vi "FOR.vi"() -> ()   [LabVIEW 2020]
panel:
  out "Numeric 2":i32
  out "Array 2":i32[](array[numeric])
  out "Array":i32[](array[numeric])
  out "Tank":u8(slide) scale=0.0..50.0
  in  "Numeric":i32
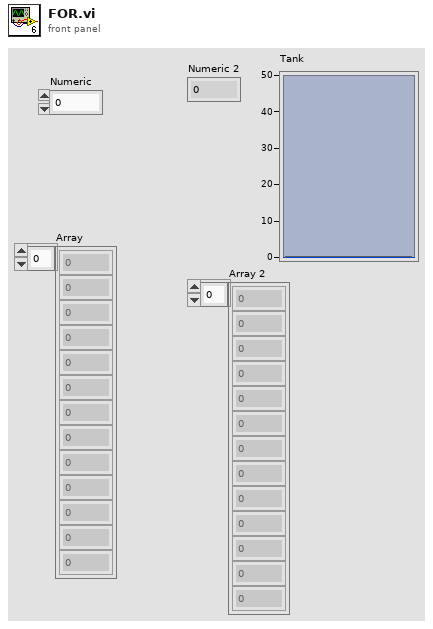
[diagram p1: front panel]
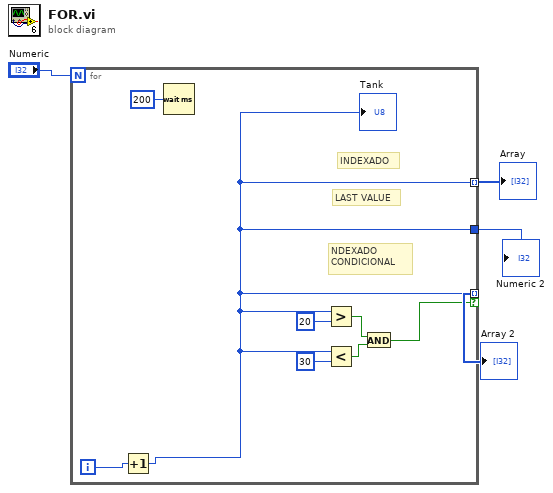
[diagram p0: block diagram]
diagram:
  n1 = for {
    N: "Numeric" -> [_]
    tunnel: [w5] -> w3 mode=indexing
    tunnel: [w5] -> w2 mode=indexing if=w8
    tunnel: [w5] -> w1
    i -> [w11]
    # "NDEXADO \nCONDICIONAL"
    # "LAST VALUE"
    # "INDEXADO"
    n2 = Increment(x=w11) -> (x+1=w5:i32)
    "Tank" <- w5
    n3 = Wait (ms)(milliseconds to wait=u32 200) -> ()  [unwired: 1 out]
    n4 = Greater?(x=w5, y=20) -> (0:w10:bool)
    n5 = Less?(x=w5, y=30) -> (x < y?=w9:bool)
    n6 = And(x=w10, y=w9) -> (x .and. y?=w8:bool)
  }
  "Array" <- w3
  "Array 2" <- w2
  "Numeric 2" <- w1
